vi "App2.vi"() -> ()   [LabVIEW 2015]
uses:
  <vilib>/DAQmx/write.llb/DAQmx Write.vi
  <vilib>/DAQmx/write.llb/DAQmx Write (Analog DBL 1Chan 1Samp).vi
  <vilib>/DAQmx/read.llb/DAQmx Read.vi
  <vilib>/DAQmx/read.llb/DAQmx Read (Analog 1D Wfm NChan NSamp).vi
  <vilib>/DAQmx/miscellaneous.llb/DAQmx Fill In Error Info.vi
panel:
  in  "stop":bool
  in  "task out":refnum<k21>
  out "Button 2":u16
  out "Waveform Chart 2":waveform(dbl)
  out "Button":u16
  in  "Tab Control":T1(tab)
  out "Vpp":dbl[](array[numeric])
  in  "Analog out":dbl(slide) scale=0.0..3.5
  out "G":dbl
  out "min value":dbl
  out "max value":dbl
  out "Delta(s)":dbl
  in  "Zero":bool
  out "Average":dbl
  out "mA/uA":bool
  out "Waveform Graph":waveform(dbl)(graph)
  in  "uA/mA":bool=TRUE
  out "Waveform Graph 2":waveform(dbl)(graph)
  out "Average (uA)":dbl caption="Average (mA)"
  in  "PAUSE":bool
  out "Vbat":dbl
  out "Waveform Chart":waveform(dbl)(graph)
  in  "USB DAQ":tag="Dev1"
  out "Waveform Graph 3":waveform(dbl)[](graph)
  in  "% Duty":i32 min=0 max=100 step=1
  in  "file List":i32(listbox)
  out "2D Picture":picture
  # "FW Validation - Current Tracking V1.0"
  # "For uC Board: 20kS/s"
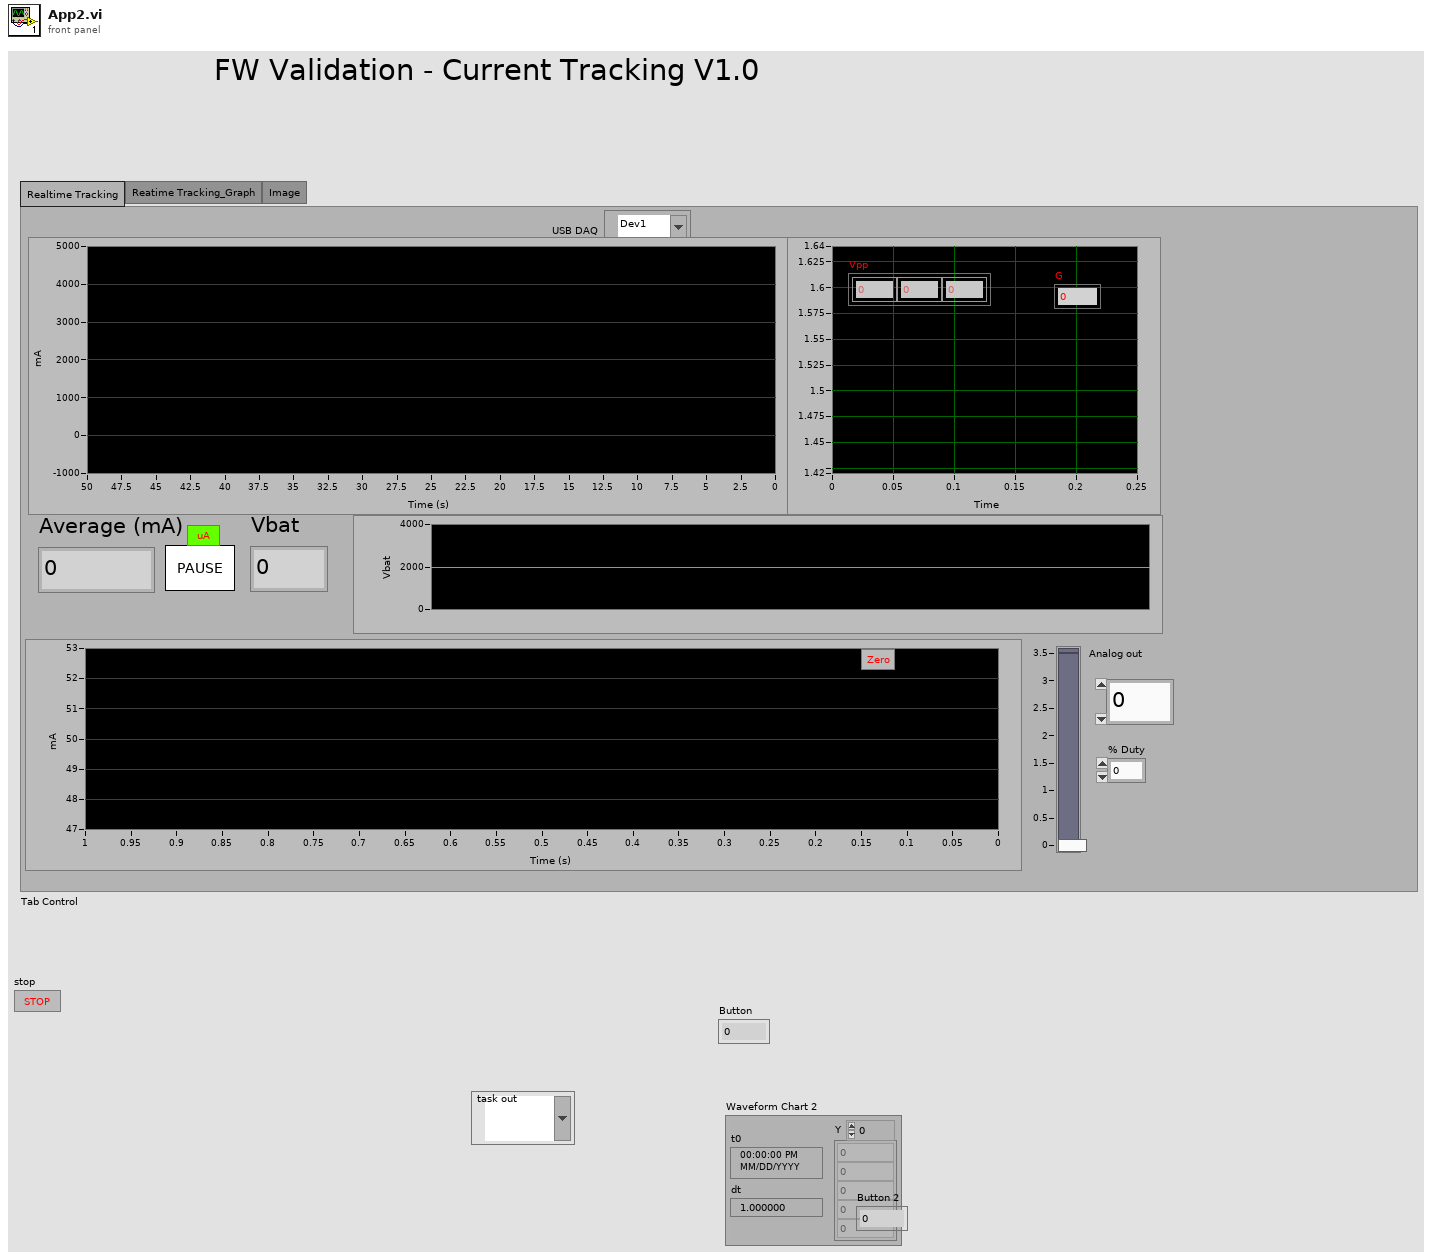
[diagram p1: front panel]
types:
  T1 = enum32{"Realtime Tracking", "Reatime Tracking_Graph", "Image"}
  T2 = typedef "imagedata.ctl" = cluster{"image type":i32, "image depth":i32, "image":u8[], "mask":u8[], "colors":u32[], "Rectangle":cluster{"left":i16, "top":i16, "right":i16, "bottom":i16}}
  T3 = typedef "LVCursorListTypeDef.ctl" = cluster{"Name":string, "Color":u32, "Style":u8, "Point Style":u8, "Name Visible":bool, "Allow Drag":bool, "Cursor Mode":u32, "Plot":i32, "Index":i32, "Position":cluster{"X":dbl, "Y":dbl}, "X Scale":u32, "Y Scale":u32, "Watch Plots":i32[], "Watch All Plots":bool, "Plot Area":i32, "Label Offset":cluster{"X":dbl, "Y":dbl}}[]
  T4 = cluster{"Name":string, "Color":u32, "Style":u8, "Point Style":u8, "Name Visible":bool, "Allow Drag":bool, "Cursor Mode":u32, "Plot":i32, "Index":i32, "Position":cluster{"X":dbl, "Y":dbl}, "X Scale":u32, "Y Scale":u32, "Watch Plots":i32[], "Watch All Plots":bool, "Plot Area":i32, "Label Offset":cluster{"X":dbl, "Y":dbl}}
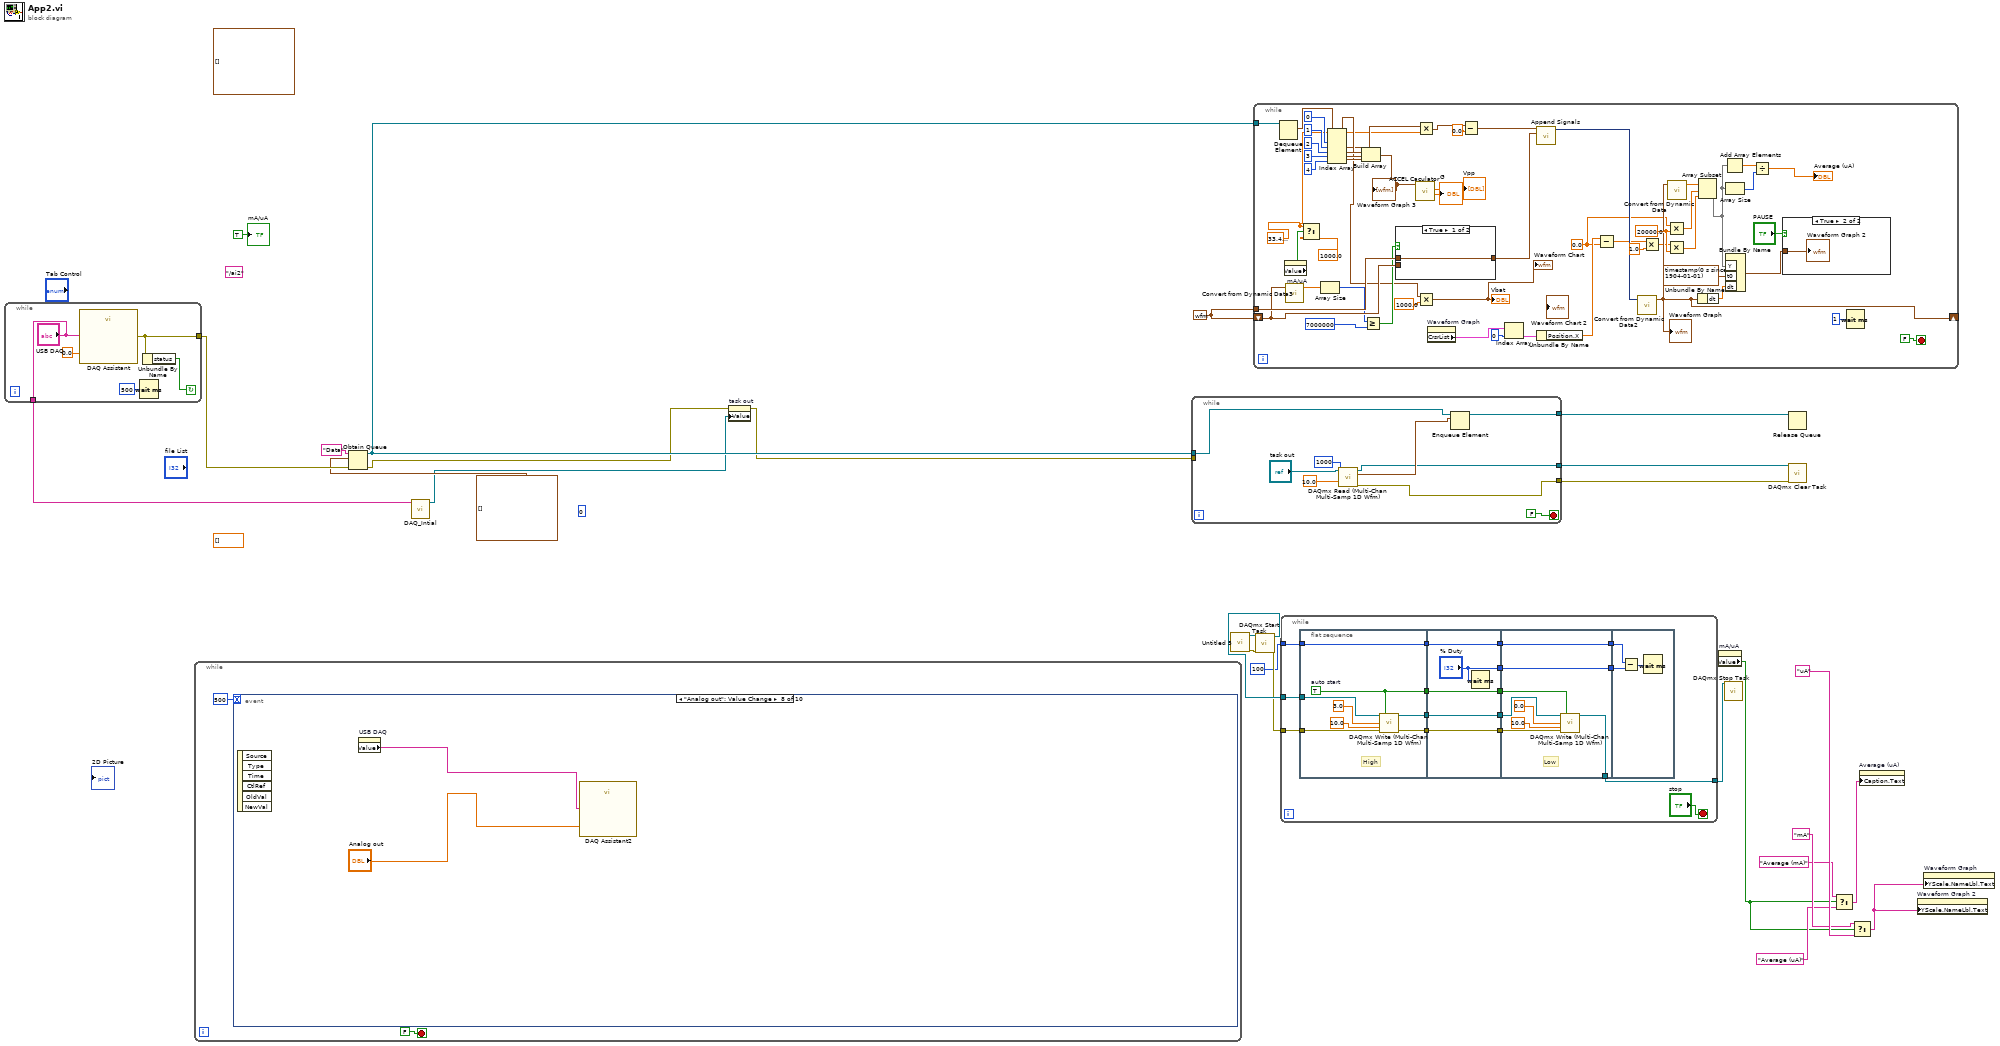
[diagram p0: block diagram]
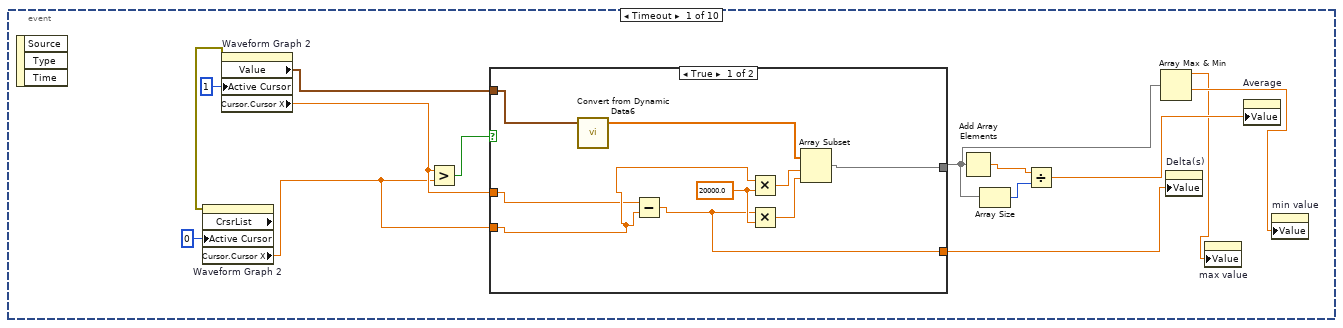
[diagram p2: hidden frame]
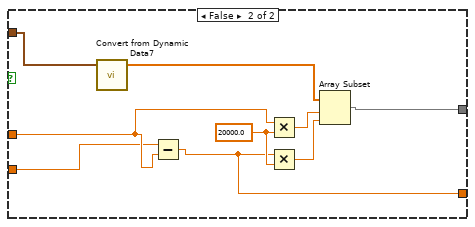
[diagram p3: hidden frame]
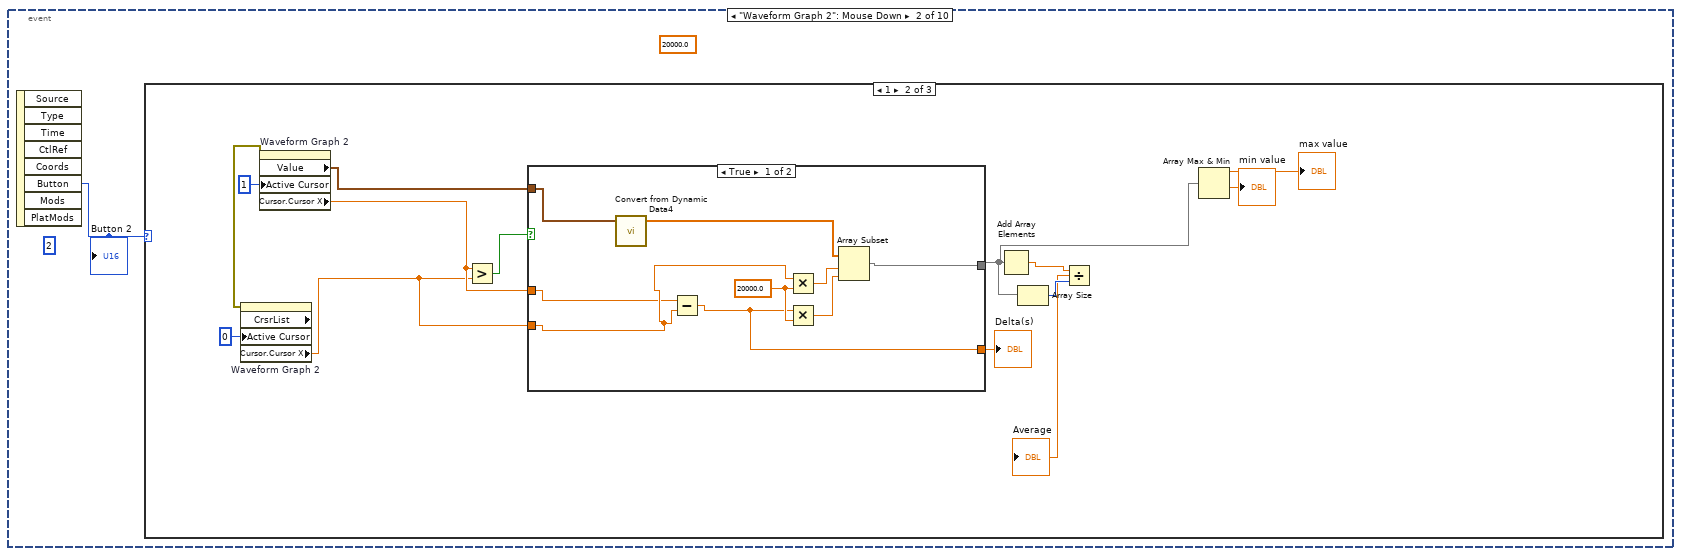
[diagram p4: hidden frame]
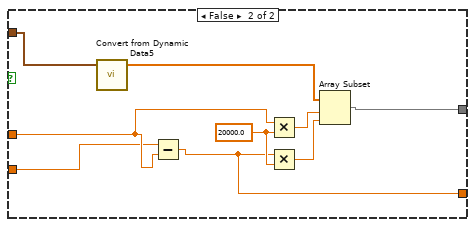
[diagram p6: hidden frame]
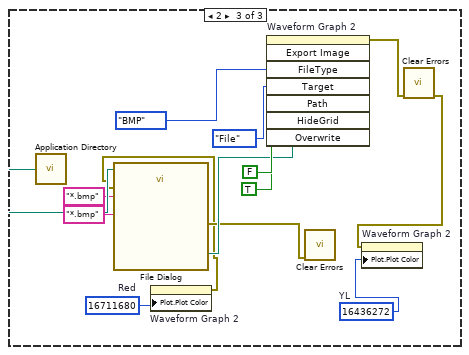
[diagram p7: hidden frame]
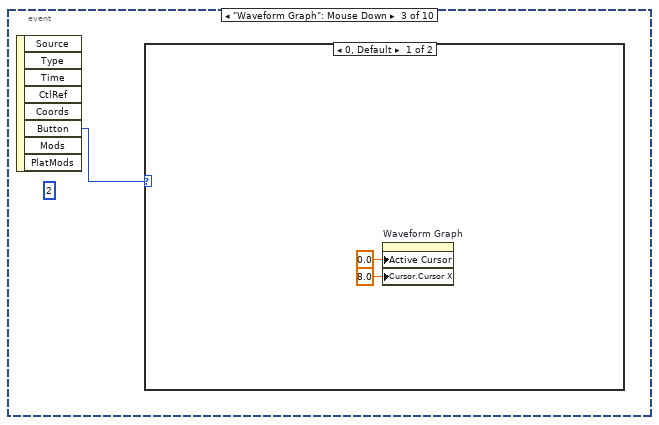
[diagram p8: hidden frame]
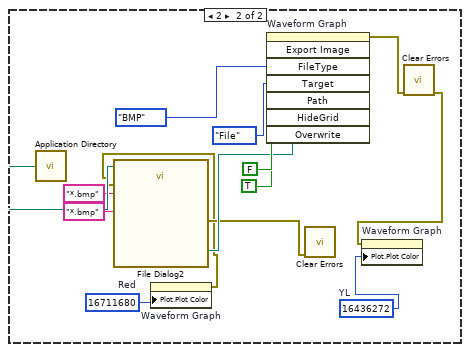
[diagram p9: hidden frame]
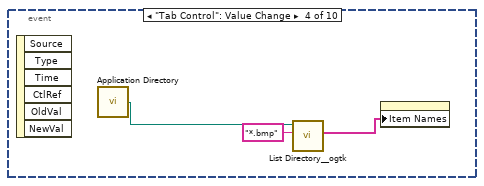
[diagram p10: hidden frame]
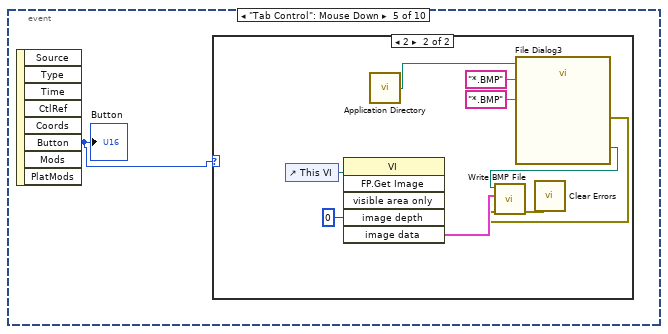
[diagram p11: hidden frame]
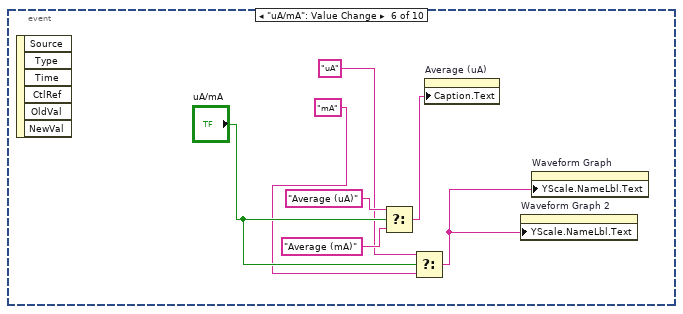
[diagram p13: hidden frame]
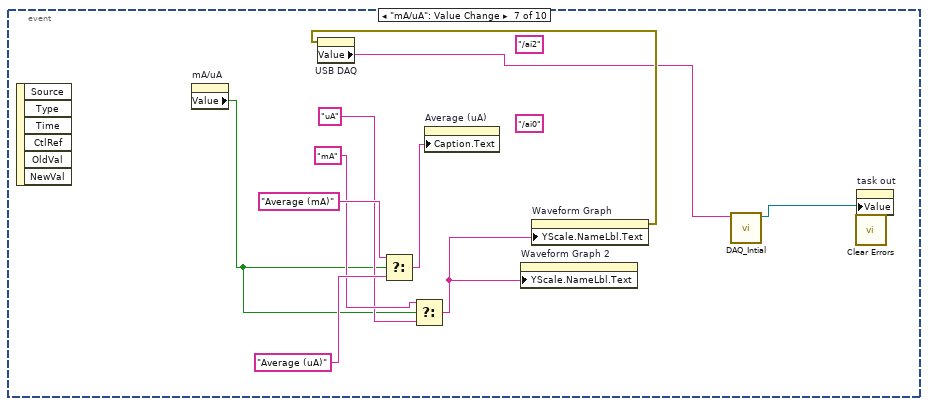
[diagram p14: hidden frame]
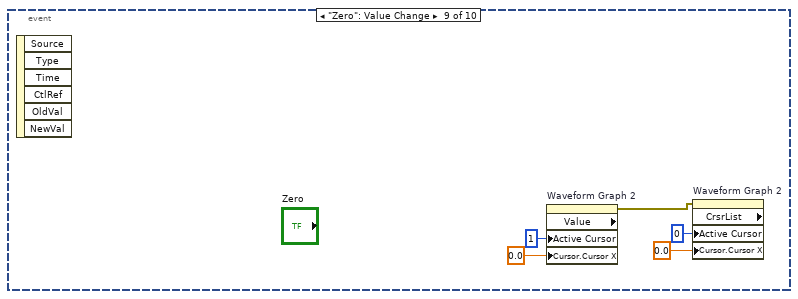
[diagram p15: hidden frame]
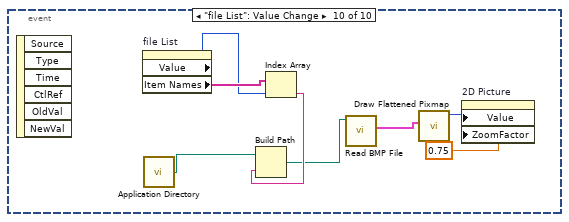
[diagram p16: hidden frame]
diagram:
  (unwired) u32 0 ("Active Cursor")
  (unwired) "/ai2" ("string")
  w21 = waveform(dbl) {"t0"=timestamp(0 s since 1904-01-01), "dt"=0.0, "Y"=[]} ("data")
  (unwired) waveform(dbl)[] [] ("History Data")
  (unwired) dbl[] [] ("Array")
  n1 = while {
    tunnel: [w29] -> w22
    tunnel: ["USB DAQ"] -> w11
    stop <- w28 continue-if-true
    n2 = call "DAQ Assistant"("data"=0.0, "device name"="USB DAQ") -> ("error out"=w29:errorcluster)  [unwired: 16 in, 1 out]
    n3 = Wait (ms)(milliseconds to wait=u32 500) -> ()  [unwired: 1 out]
    n4 = Unbundle By Name(w29) -> ("status"=w28:bool)
  }
  n5 = while {
    stop <- FALSE stop-if-true
    n6 = event shown="[7] \"Analog out\": Value Change" {
      selector: _ -> [_ _ _ _ _ _ _ _ _ _]
      dyn-events: _ -> [_ _ _ _ _ _ _ _ _ _]
      timeout: 500 -> [_ _ _ _ _ _ _ _ _ _]
      event Timeout {
        n7 = event-data() -> ()  [unwired: 1 in, 3 out]
        n8 = property on="Waveform Graph 2" class="WFGraph (strict)"("Active Cursor"=u32 1) -> (error out=w42:errorcluster, "Value"=w38:waveform(dbl), "Cursor.Cursor X"=w44:dbl)  [unwired: 2 in, 1 out]
        n9 = property on="Waveform Graph 2" class="WFGraph (strict)" props=["CrsrList", "Active Cursor", "Cursor", "Cursor X"](error in=w42, "Active Cursor"=u32 0) -> ("Cursor.Cursor X"=w43:dbl)  [unwired: 1 in, 3 out]
        n10 = Greater?(x=w44, y=w43) -> (0:w45:bool)
        n11 = case shown="True" w45 {
          tunnel: w38 -> [w56 w65]
          tunnel: w44 -> [w49 w59]
          tunnel: w43 -> [w50 w58]
          tunnel: [w51 w60] -> w39
          tunnel: [w48 w57] -> w37
          frame True {
            w54 = 20000.0 ("y")
            n12 = call "Convert from Dynamic Data6"("Dynamic Data Type"=w56) -> ("Array"=w52:dbl[])  [unwired: 3 in]
            n13 = Subtract(x=w49, y=w50) -> (x-y=w48:dbl)
            n14 = Multiply(x=w50, y=w54) -> (x*y=w55:dbl)
            n15 = Multiply(x=w48, y=w54) -> (x*y=w53:dbl)
            n16 = Array Subset(array=w52, index=w55, length=w53) -> (w51:dbl[])
          }
          frame False {
            w63 = 20000.0 ("y")
            n17 = call "Convert from Dynamic Data7"("Dynamic Data Type"=w65) -> ("Array"=w61:dbl[])  [unwired: 3 in]
            n18 = Subtract(x=w58, y=w59) -> (x-y=w57:dbl)
            n19 = Multiply(x=w59, y=w63) -> (x*y=w64:dbl)
            n20 = Multiply(x=w57, y=w63) -> (x*y=w62:dbl)
            n21 = Array Subset(array=w61, index=w64, length=w62) -> (w60:dbl[])
          }
        }
        n22 = Add Array Elements(numeric array=w39) -> (sum=w41:dbl)
        n23 = Array Size(array=w39) -> (size(s)=w40:i32)
        n24 = Divide(x=w41, y=w40) -> (x/y=w36:dbl)
        n25 = Array Max & Min(array=w39) -> (max value=w34:dbl, min value=w35:dbl)  [unwired: 2 out]
        n26 = property on="Delta(s)" class="DigNum (strict)"("Value"=w37) -> ()  [unwired: 2 in, 2 out]
        n27 = property on="max value" class="DigNum (strict)"("Value"=w34) -> ()  [unwired: 2 in, 2 out]
        n28 = property on="Average" class="DigNum (strict)"("Value"=w36) -> ()  [unwired: 2 in, 2 out]
        n29 = property on="min value" class="DigNum (strict)"("Value"=w35) -> ()  [unwired: 2 in, 2 out]
      }
      event "Waveform Graph 2": Mouse Down {
        (unwired) 20000.0 ("y")
        (unwired) u16 2 ("Button")
        n30 = event-data() -> ("Button"=w66:u16)  [unwired: 1 in, 7 out]
        "Button 2" <- w66
        n31 = case shown="1" w66 {
          frame 0, Default {
          }
          frame 1 {
            n32 = property on="Waveform Graph 2" class="WFGraph (strict)"("Active Cursor"=u32 1) -> (error out=w75:errorcluster, "Value"=w67:waveform(dbl), "Cursor.Cursor X"=w77:dbl)  [unwired: 2 in, 1 out]
            n33 = property on="Waveform Graph 2" class="WFGraph (strict)" props=["CrsrList", "Active Cursor", "Cursor", "Cursor X"](error in=w75, "Active Cursor"=u32 0) -> ("Cursor.Cursor X"=w76:dbl)  [unwired: 1 in, 3 out]
            n34 = Greater?(x=w77, y=w76) -> (0:w78:bool)
            n35 = case shown="True" w78 {
              tunnel: w67 -> [w89 w98]
              tunnel: w77 -> [w82 w92]
              tunnel: w76 -> [w83 w91]
              tunnel: [w84 w93] -> w70
              tunnel: [w81 w90] -> w71
              frame True {
                w87 = 20000.0 ("y")
                n36 = call "Convert from Dynamic Data4"("Dynamic Data Type"=w89) -> ("Array"=w85:dbl[])  [unwired: 3 in]
                n37 = Subtract(x=w82, y=w83) -> (x-y=w81:dbl)
                n38 = Multiply(x=w83, y=w87) -> (x*y=w88:dbl)
                n39 = Multiply(x=w81, y=w87) -> (x*y=w86:dbl)
                n40 = Array Subset(array=w85, index=w88, length=w86) -> (w84:dbl[])
              }
              frame False {
                w96 = 20000.0 ("y")
                n41 = call "Convert from Dynamic Data5"("Dynamic Data Type"=w98) -> ("Array"=w94:dbl[])  [unwired: 3 in]
                n42 = Subtract(x=w91, y=w92) -> (x-y=w90:dbl)
                n43 = Multiply(x=w92, y=w96) -> (x*y=w97:dbl)
                n44 = Multiply(x=w90, y=w96) -> (x*y=w95:dbl)
                n45 = Array Subset(array=w94, index=w97, length=w95) -> (w93:dbl[])
              }
            }
            "Delta(s)" <- w71
            n46 = Add Array Elements(numeric array=w70) -> (sum=w74:dbl)
            n47 = Array Size(array=w70) -> (size(s)=w73:i32)
            n48 = Divide(x=w74, y=w73) -> (x/y=→"Average":dbl)
            n49 = Array Max & Min(array=w70) -> (max value=→"max value":dbl, min value=→"min value":dbl)  [unwired: 2 out]
          }
          frame 2 {
            w99 = u32 16436272  # YL
            w101 = u32 16711680  # Red
            n50 = call <vilib>:"Application Directory.vi"() -> ("Application Directory"=w108:path)
            n51 = property on="Waveform Graph 2" class="WFGraph (strict)"("Plot.Plot Color"=w101) -> (error out=w102:errorcluster)  [unwired: 2 in, 1 out]
            n52 = call "File Dialog"("start path"=w108, "error in"=w102, "pattern (all files)"="*.bmp", "pattern label"="*.bmp") -> ("selected path"=w105:path, "error out"=w104:errorcluster)  [unwired: 8 in, 2 out]
            n53 = invoke on="Waveform Graph 2" class="WFGraph (strict)" method="Export Image"("FileType"=enum32{"BMP", "EPS", "EMF", "PICT"}."BMP" ("File Type"), "Target"=enum32{"File", "Clipboard"}."File", "Path"=w105, "HideGrid"=FALSE ("Hide Grid"), "Overwrite"=TRUE ("Always Overwrite")) -> (error out=w103:errorcluster)  [unwired: 3 in, 7 out]
            n54 = call <vilib>:"Clear Errors.vi"("error in (no error)"=w104) -> ()  [unwired: 5 in, 2 out]
            n55 = call <vilib>:"Clear Errors.vi"("error in (no error)"=w103) -> ("error out"=w100:errorcluster)  [unwired: 5 in, 1 out]
            n56 = property on="Waveform Graph 2" class="WFGraph (strict)"(error in=w100, "Plot.Plot Color"=w99) -> ()  [unwired: 1 in, 2 out]
          }
        }
      }
      event "Waveform Graph": Mouse Down {
        (unwired) u16 2 ("Button")
        n57 = event-data() -> ("Button"=w113:u16)  [unwired: 1 in, 7 out]
        n58 = case shown="0, Default" w113 {
          frame 0, Default {
            n59 = property on="Waveform Graph" class="WFGraph (strict)"("Active Cursor"=0.0 ("Cursor.Cursor Position:Cursor X"), "Cursor.Cursor X"=8.0 ("Cursor.Cursor Position:Cursor X")) -> ()  [unwired: 2 in, 2 out]
          }
          frame 2 {
            w116 = u32 16436272  # YL
            w118 = u32 16711680  # Red
            n60 = call <vilib>:"Application Directory.vi"() -> ("Application Directory"=w125:path)
            n61 = property on="Waveform Graph" class="WFGraph (strict)"("Plot.Plot Color"=w118) -> (error out=w119:errorcluster)  [unwired: 2 in, 1 out]
            n62 = call "File Dialog2"("start path"=w125, "error in"=w119, "pattern (all files)"="*.bmp", "pattern label"="*.bmp") -> ("selected path"=w122:path, "error out"=w121:errorcluster)  [unwired: 8 in, 2 out]
            n63 = invoke on="Waveform Graph" class="WFGraph (strict)" method="Export Image"("FileType"=enum32{"BMP", "EPS", "EMF", "PICT"}."BMP" ("File Type"), "Target"=enum32{"File", "Clipboard"}."File", "Path"=w122, "HideGrid"=FALSE ("Hide Grid"), "Overwrite"=TRUE ("Always Overwrite")) -> (error out=w120:errorcluster)  [unwired: 3 in, 7 out]
            n64 = call <vilib>:"Clear Errors.vi"("error in (no error)"=w121) -> ()  [unwired: 5 in, 2 out]
            n65 = call <vilib>:"Clear Errors.vi"("error in (no error)"=w120) -> ("error out"=w117:errorcluster)  [unwired: 5 in, 1 out]
            n66 = property on="Waveform Graph" class="WFGraph (strict)"(error in=w117, "Plot.Plot Color"=w116) -> ()  [unwired: 1 in, 2 out]
          }
        }
      }
      event "Tab Control": Value Change {
        n67 = event-data() -> ()  [unwired: 1 in, 6 out]
        n68 = call <vilib>:"Application Directory.vi"() -> ("Application Directory"=w132:path)
        n69 = call <userlib>:"List Directory__ogtk.vi"("pattern"="*.bmp", "directory path"=w132) -> ("file names"=w130:string[])  [unwired: 2 in, 3 out]
        n70 = property on="file List" class="LstBox (strict)"("Item Names"=w130) -> ()  [unwired: 2 in, 2 out]
      }
      event "Tab Control": Mouse Down {
        n71 = event-data() -> ("Button"=w133:u16)  [unwired: 1 in, 7 out]
        "Button" <- w133
        n72 = case shown="2" w133 {
          frame 0, Default {
          }
          frame 2 {
            n73 = control-ref of="This VI"() -> (w142:refnum<vi>)
            n74 = invoke class="VI" method="FP.Get Image"(reference=w142, "image depth"=0 ("Image Depth")) -> ("image data"=w140:T2)  [unwired: 4 in, 5 out]
            n75 = call <vilib>:"Application Directory.vi"() -> ("Application Directory"=w136:path)
            n76 = call "File Dialog3"("start path"=w136, "pattern (all files)"="*.BMP", "pattern label"="*.BMP") -> ("selected path"=w139:path, "error out"=w138:errorcluster)  [unwired: 9 in, 2 out]
            n77 = call <vilib>:"Write BMP File.vi"("error in (no error)"=w138, "image data"=w140, "path to BMP file"=w139) -> ("error out"=w134:errorcluster)  [unwired: 7 in, 1 out]
            n78 = call <vilib>:"Clear Errors.vi"("error in (no error)"=w134) -> ()  [unwired: 5 in, 2 out]
          }
        }
      }
      event "uA/mA": Value Change {
        n79 = event-data() -> ()  [unwired: 1 in, 6 out]
        n80 = Select(t="Average (uA)" ("Caption.Text"), s="uA/mA", f="Average (mA)" ("Caption.Text")) -> (s? t:f=w149:string)
        n81 = Select(t="uA" ("Caption.Text"), s="uA/mA", f="mA" ("Caption.Text")) -> (s? t:f=w143:string)
        n82 = property on="Average (uA)" class="DigNum (strict)"("Caption.Text"=w149) -> ()  [unwired: 2 in, 2 out]
        n83 = property on="Waveform Graph 2" class="WFGraph (strict)"("YScale.NameLbl.Text"=w143) -> ()  [unwired: 2 in, 2 out]
        n84 = property on="Waveform Graph" class="WFGraph (strict)"("YScale.NameLbl.Text"=w143) -> ()  [unwired: 2 in, 2 out]
      }
      event "mA/uA": Value Change {
        (unwired) "/ai0" ("string")
        (unwired) "/ai2" ("string")
        n85 = event-data() -> ()  [unwired: 1 in, 6 out]
        n86 = property on="mA/uA" class="Bool (strict)"() -> ("Value"=w153:bool)  [unwired: 2 in, 2 out]
        n87 = Select(t="Average (mA)" ("Caption.Text"), s=w153, f="Average (uA)" ("Caption.Text")) -> (s? t:f=w159:string)
        n88 = Select(t="mA" ("Caption.Text"), s=w153, f="uA" ("Caption.Text")) -> (s? t:f=w158:string)
        n89 = property on="Average (uA)" class="DigNum (strict)"("Caption.Text"=w159) -> ()  [unwired: 2 in, 2 out]
        n90 = property on="Waveform Graph 2" class="WFGraph (strict)"("YScale.NameLbl.Text"=w158) -> ()  [unwired: 2 in, 2 out]
        n91 = property on="Waveform Graph" class="WFGraph (strict)"("YScale.NameLbl.Text"=w158) -> (error out=w152:errorcluster)  [unwired: 2 in, 1 out]
        n92 = property on="USB DAQ" class="DAQmxName"(error in=w152) -> ("Value"=w151:string)  [unwired: 1 in, 2 out]
        n93 = call "DAQ_Intial.vi"("DEV"=w151) -> ("task out"=w150:refnum<k21>)  [unwired: 9 in, 1 out]
        n94 = call <vilib>:"Clear Errors.vi"() -> ()  [unwired: 6 in, 2 out]
        n95 = property on="task out" class="DAQmxName (strict)"("Value"=w150) -> ()  [unwired: 2 in, 2 out]
      }
      event "Analog out": Value Change {
        n96 = event-data() -> ()  [unwired: 1 in, 6 out]
        n97 = property on="USB DAQ" class="DAQmxName"() -> ("Value"=w161:string)  [unwired: 2 in, 2 out]
        n98 = call "DAQ Assistant2"("data"="Analog out", "device name"=w161) -> ()  [unwired: 16 in, 2 out]
      }
      event "Zero": Value Change {
        n99 = event-data() -> ()  [unwired: 1 in, 6 out]
        n100 = property on="Waveform Graph 2" class="WFGraph (strict)" props=["Value", "Active Cursor", "Cursor", "Cursor X"]("Active Cursor"=u32 1, "Cursor.Cursor X"=0.0 ("Cursor.Cursor Position:Cursor X")) -> (error out=w164:errorcluster)  [unwired: 2 in, 2 out]
        n101 = property on="Waveform Graph 2" class="WFGraph (strict)" props=["CrsrList", "Active Cursor", "Cursor", "Cursor X"](error in=w164, "Active Cursor"=u32 0, "Cursor.Cursor X"=0.0 ("Cursor.Cursor Position:Cursor X")) -> ()  [unwired: 1 in, 3 out]
      }
      event "file List": Value Change {
        n102 = event-data() -> ()  [unwired: 1 in, 6 out]
        n103 = property on="file List" class="LstBox (strict)"() -> ("Value"=w173:i32, "Item Names"=w174:string[])  [unwired: 2 in, 2 out]
        n104 = call <vilib>:"Application Directory.vi"() -> ("Application Directory"=w170:path)
        n105 = Index Array(array=w174, index=w173) -> (element=w169:string)
        n106 = Build Path(base path=w170, name or relative path=w169) -> (appended path=w168:path)
        n107 = call <vilib>:"Read BMP File.vi"("path to BMP file"=w168) -> ("image data"=w172:T2)  [unwired: 8 in, 2 out]
        n108 = call <vilib>:"Draw Flattened Pixmap.vi"("image data"=w172) -> ("new picture"=w171:picture)  [unwired: 8 in]
        n109 = property on="2D Picture" class="Pict"("Value"=w171, "ZoomFactor"=sgl 0.75 ("Zoom Factor")) -> ()  [unwired: 2 in, 2 out]
      }
    }
  }
  n110 = Obtain Queue(name (unnamed)="Data", element data type=waveform(dbl)[] [] ("data"), error in (no error)=w22) -> (queue out=w24:refnum<queue>, error out=w13:errorcluster)  [unwired: 2 in, 1 out]
  n111 = call "DAQ_Intial.vi"("DEV"=w11) -> ("task out"=w9:refnum<k21>)  [unwired: 9 in, 1 out]
  n112 = property on="task out" class="DAQmxName (strict)"(error in=w13, "Value"=w9) -> (error out=w12:errorcluster)  [unwired: 1 in, 1 out]
  n113 = while {
    tunnel: [w180] -> w26
    tunnel: w24 -> [w183]
    tunnel: [w182] -> w23
    tunnel: w12 -> [_]
    tunnel: [w175] -> w8
    stop <- FALSE ("stop (F)") stop-if-true
    n114 = call-poly "DAQmx Read (Multi-Chan Multi-Samp 1D Wfm).vi"("task/channels in"="task out", "number of samples per channel"=1000, "timeout"=10.0) -> ("task out"=w175:refnum<k21>, "data"=w176:waveform(dbl)[], "error out"=w180:errorcluster)  [unwired: 10 in]
    n115 = Enqueue Element(queue=w183, element=w176) -> (queue out=w182:refnum<queue>)  [unwired: 2 in, 2 out]
  }
  n116 = call "Untitled 5.vi"() -> ("error out"=w5:errorcluster, "task out"=w6:refnum<k21>)  [unwired: 10 in]
  n117 = while {
    tunnel: w24 -> [w237]
    shift-right: [w226] -> _
    shift-left: w21 -> [w209]
    tunnel: w21 -> [w210]
    stop <- FALSE stop-if-true
    w185 = 33.499999999999986 ("y")
    w216 = 0.0
    w230 = 20000.0 ("y")
    n118 = Dequeue Element(queue=w237) -> (element=w198:waveform(dbl)[])  [unwired: 2 in, 3 out]
    n119 = property on="mA/uA" class="Bool (strict)"() -> ("Value"=w201:bool)  [unwired: 2 in, 2 out]
    n120 = call "Convert from Dynamic Data3"("Dynamic Data Type"=w209) -> ("Array"=w208:dbl[])  [unwired: 3 in]
    n121 = Select(t=w185, s=w201, f=1000.0 ("y")) -> ()  [unwired: 1 out]
    n122 = Array Size(array=w208) -> (size(s)=w207:i32)
    n123 = Index Array(array=w198, index #1=0 ("index"), index #2=1 ("index"), index #3=2 ("index"), index #4=3 ("index"), index #5=4 ("index")) -> (element #1=w187:waveform(dbl), element #2=w186:waveform(dbl), element #3=w192:waveform(dbl), element #4=w191:waveform(dbl), element #5=w190:waveform(dbl))
    n124 = Build Array(w192, w191, w190) -> (w189:waveform(dbl)[])
    "Waveform Graph 3" <- w189
    n125 = Greater Or Equal?(x=w207, y=7000000 ("size(s)")) -> (x >= y?=w205:bool)
    n126 = case shown="True" w205 {
      tunnel: w209 -> [_ w239]
      tunnel: [w238 w239] -> w211
      tunnel: w210 -> [w238 _]
      frame True {
      }
      frame False {
      }
    }
    n127 = call "ACCEL Caculator.vi"("appended array"=w189) -> ("Result"=→"G":dbl, "Array"=→"Vpp":dbl[])  [unwired: 7 in, 2 out]
    n128 = Multiply(x=w186, y=w185) -> (x*y=w202:waveform(dbl))
    n129 = Multiply(x=w187, y=1000.0) -> (x*y=→"Vbat" →"Waveform Chart":waveform(dbl))
    n130 = property on="Waveform Graph" class="WFGraph (strict)"() -> ("CrsrList"=w233:T3)  [unwired: 2 in, 2 out]
    n131 = Subtract(x=w202, y=0.0) -> (x-y=w203:waveform(dbl))
    n132 = Index Array(array=w233, index=0) -> (element=w214:T4)
    n133 = call "Append Signals"("Input Signal B"=w211, "Input Signal A"=w203) -> ("Appended Signals"=w234:dynamicdata)  [unwired: 8 in, 1 out]
    n134 = Unbundle By Name(w214) -> ("Position.X"=w217:dbl)
    n135 = Subtract(x=w217, y=w216) -> (x-y=w220:dbl)
    n136 = call "Convert from Dynamic Data2"("Dynamic Data Type"=w234) -> ("Waveform"=w226:waveform(dbl))  [unwired: 3 in]
    "Waveform Graph" <- w226
    n137 = Multiply(x=w220, y=1.0) -> (x*y=w218:dbl)
    n138 = Multiply(x=w216, y=w230) -> (x*y=w231:dbl)
    n139 = Multiply(x=w218, y=w230) -> (x*y=w229:dbl)
    n140 = call "Convert from Dynamic Data"("Dynamic Data Type"=w226) -> ("Array"=w199:dbl[])  [unwired: 3 in]
    n141 = Unbundle By Name(w226) -> ("dt"=w225:dbl)
    n142 = Array Subset(array=w199, index=w231, length=w229) -> (w224:dbl[])
    n143 = Add Array Elements(numeric array=w224) -> (sum=w223:dbl)
    n144 = Bundle By Name("Y"=w224, "t0"=timestamp(0 s since 1904-01-01), "dt"=w225) -> (w228:waveform(dbl))  [unwired: 1 in]
    n145 = Array Size(array=w224) -> (size(s)=w222:i32)
    n146 = Divide(x=w223, y=w222) -> (x/y=→"Average (uA)":dbl)
    n147 = case shown="True" "PAUSE" {
      tunnel: w228 -> [_ w240]
      frame False {
      }
      frame True {
        "Waveform Graph 2" <- w240
      }
    }
    n148 = Wait (ms)(milliseconds to wait=u32 1) -> ()  [unwired: 1 out]
  }
  n149 = call <vilib>:"DAQmx Start Task.vi"("task/channels in"=w6, "error in"=w5) -> ("task out"=w4:refnum<k21>, "error out"=w3:errorcluster)  [unwired: 12 in]
  n150 = while {
    tunnel: w4 -> [w245]
    tunnel: w3 -> [w241]
    tunnel: 100 -> [w253]
    tunnel: [w244] -> w1
    stop <- "stop" stop-if-true
    n151 = flat-sequence {
      tunnel: [w264] -> w256
      tunnel: w253 -> [w263]
      tunnel: [w263] -> w251
      tunnel: [w261] -> w247
      tunnel: w245 -> [w260]
      tunnel: [w259] -> w243
      tunnel: w241 -> [w258]
      tunnel: w256 -> [w269]
      tunnel: [w269] -> w255
      tunnel: [w268] -> w252
      tunnel: w251 -> [w268]
      tunnel: ["% Duty"] -> w249
      tunnel: w247 -> [w266]
      tunnel: [w266] -> w246
      tunnel: w243 -> [w265]
      tunnel: [w265] -> w242
      tunnel: w255 -> [w277]
      tunnel: w252 -> [w276]
      tunnel: [w276] -> w250
      tunnel: w249 -> [w275]
      tunnel: [w275] -> w248
      tunnel: w246 -> [w273]
      tunnel: [w272] -> w244
      tunnel: w242 -> [w271]
      tunnel: w250 -> [w280]
      tunnel: w248 -> [w279]
      frame #0 {
        w264 = TRUE  # auto start
        # "High"
        n152 = call-poly "DAQmx Write (Multi-Chan Multi-Samp 1D Wfm).vi"("task/channels in"=w260, "auto start"=w264, "data"=3.0, "timeout"=10.0, "error in"=w258) -> ("task out"=w261:refnum<k21>, "error out"=w259:errorcluster)  [unwired: 8 in, 1 out]
      }
      frame #1 {
        n153 = Wait (ms)(milliseconds to wait="% Duty") -> ()  [unwired: 1 out]
      }
      frame #2 {
        # "Low"
        n154 = call-poly "DAQmx Write (Multi-Chan Multi-Samp 1D Wfm).vi"("task/channels in"=w273, "auto start"=w277, "data"=0.0, "timeout"=10.0, "error in"=w271) -> ("task out"=w272:refnum<k21>)  [unwired: 8 in, 2 out]
      }
      frame #3 {
        n155 = Subtract(x=w280, y=w279) -> (x-y=w278:i32)
        n156 = Wait (ms)(milliseconds to wait=w278) -> ()  [unwired: 1 out]
      }
    }
  }
  n157 = property on="mA/uA" class="Bool (strict)"() -> ("Value"=w16:bool)  [unwired: 2 in, 2 out]
  n158 = call <vilib>:"DAQmx Stop Task.vi"("task/channels in"=w1) -> ()  [unwired: 13 in, 2 out]
  n159 = Release Queue(queue=w23) -> ()  [unwired: 2 in, 3 out]
  n160 = call <vilib>:"DAQmx Clear Task.vi"("task in"=w8, "error in"=w26) -> ()  [unwired: 13 in, 1 out]
  n161 = Select(t="Average (mA)" ("Caption.Text"), s=w16, f="Average (uA)" ("Caption.Text")) -> (s? t:f=w14:string)
  n162 = Select(t="mA" ("Caption.Text"), s=w16, f="uA" ("Caption.Text")) -> (s? t:f=w15:string)
  n163 = property on="Average (uA)" class="DigNum (strict)"("Caption.Text"=w14) -> ()  [unwired: 2 in, 2 out]
  n164 = property on="Waveform Graph 2" class="WFGraph (strict)"("YScale.NameLbl.Text"=w15) -> ()  [unwired: 2 in, 2 out]
  n165 = property on="Waveform Graph" class="WFGraph (strict)"("YScale.NameLbl.Text"=w15) -> ()  [unwired: 2 in, 2 out]
  "mA/uA" <- TRUE ("mA/uA")
